vi "FIR Windowed Filter (CDB).vi"(0 "sampling freq: fs":dbl=1.0 format="%0.2f", 1 "X":cdb[](array[numeric]), 2 "filter type":T2, 3 "window parameter":dbl=nan, 7 "low cutoff freq: fl":dbl=0.125 format="%0.2f", 11 "high cutoff freq: fh":dbl=0.45 format="%0.2f", 12 "taps":i32=25 min=1, 14 "window":T1 items=["Rectangle"=0, "Hanning"=1, "Hamming"=2, "Blackman-Harris"=3, "Exact Blackman"=4, "Blackman"=5, "Flat Top"=6, "4 Term B-Harris "=7, "7 Term B-Harris"=8, "Low Sidelobe"=9, "Blackman Nuttall"=11, "Triangle"=30, "Bartlett-Hanning"=31, "Bohman"=32, "Parzen"=33, "Welch"=34, "Kaiser"=60, "Dolph-Chebyshev"=61, "Gaussian"=62]) -> (4 "Filtered X":cdb[](array[numeric]), 10 "error":i32)   [LabVIEW 2020, in "NI_AALBase.lvlib"]
doc: "Filters the input data sequence, <B>X</B>, using the set of windowed FIR filter coefficients specified by the <B>sampling freq: fs</B>, <B>low cutoff freq: fl</B>, <B>high cutoff freq: fh</B>, and number of <B>taps</B>. Wire data to the <B>X</B> input to determine the polymorphic instance to use or manually select the instance."
uses:
  NI_AALBase.lvlib
  Filter Passband Type.ctl
  windowTd.ctl
  1D Convolution (DBL).vi
  NI_AALPro.lvlib
panel:
  # "FIR Windowed Filter"
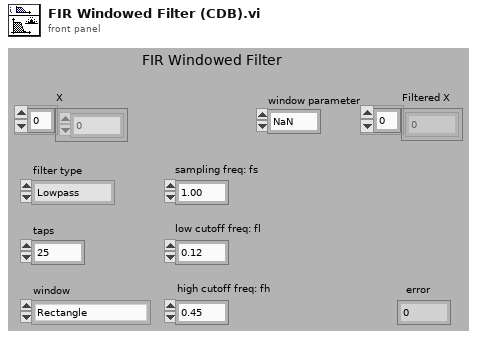
[diagram p1: front panel]
types:
  T1 = typedef "NI_AALPro.lvlib/windowTd.ctl" = u32
  T2 = typedef "NI_AALBase.lvlib/Filter Passband Type.ctl" = enum32{"Lowpass", "Highpass", "Bandpass", "Bandstop"}
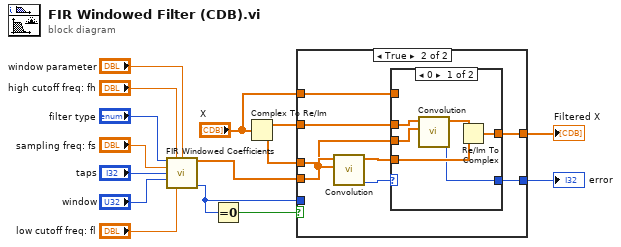
[diagram p0: block diagram]
diagram:
  n1 = call "FIR Windowed Coefficients.vi"("filter type"="filter type", "high cutoff freq: fh"="high cutoff freq: fh", "window parameter"="window parameter", "sampling freq: fs"="sampling freq: fs", "taps"="taps", "window"="window", "low cutoff freq: fl"="low cutoff freq: fl") -> ("FIR Windowed Coefficients"=w7:dbl[], "error"=w8:i32)  [unwired: 1 in, 6 out]
  n2 = Equal To 0?(x=w8) -> (x = 0?=w9:bool)
  n3 = Complex To Re/Im(x + iy="X") -> (x=w6:dbl[], y=w5:dbl[])
  n4 = case shown="True" w9 {
    tunnel: w8 -> [w17 _]
    tunnel: [w17 w19] -> w3
    tunnel: [w16 w21] -> w4
    tunnel: w5 -> [_ w25]
    tunnel: w7 -> [_ w22]
    tunnel: w6 -> [_ w23]
    tunnel: "X" -> [w16 w18]
    frame False {
    }
    frame True {
      n5 = call-poly "Convolution.vi"("Y"=w22, "X"=w25) -> ("error"=w24:i32, "X * Y"=w20:dbl[])  [unwired: 1 in, 7 out]
      n6 = case shown="0" w24 {
        selector: w24 -> [_ w33]
        tunnel: w23 -> [w31 _]
        tunnel: w22 -> [w30 _]
        tunnel: [w28 w32] -> w21
        tunnel: w20 -> [w29 _]
        tunnel: [w27 w33] -> w19
        tunnel: w18 -> [_ w32]
        frame 0 {
          n7 = call-poly "Convolution.vi"("Y"=w30, "X"=w31) -> ("error"=w27:i32, "X * Y"=w26:dbl[])  [unwired: 1 in, 7 out]
          n8 = Re/Im To Complex(1:w29, 2:w26) -> (0:w28:cdb[])
        }
        frame Default {
        }
      }
    }
  }
  "Filtered X" <- w4
  "error" <- w3
